vi "test-cubic-spline-04A.vi"() -> (3 "Test Passed":bool)   [LabVIEW 2019]
uses:
  <vilib>/Rock Robotics/WPI/ThirdParty/JAS_Junk/TrajLib/POSEwCURVATURE.ctl
  <vilib>/Rock Robotics/WPI/ThirdParty/JAS_Junk/TrajLib/POSE2D.ctl
  <vilib>/Rock Robotics/WPI/ThirdParty/JAS_Junk/TrajLib/TRANSLATION2D.ctl
  <vilib>/Rock Robotics/WPI/ThirdParty/JAS_Junk/TrajLib/ROTATION2D.ctl
  <vilib>/Rock Robotics/WPI/ThirdParty/JAS_Junk/TrajLib/Rotation_CreateAngle.vi
  <vilib>/Rock Robotics/WPI/ThirdParty/JAS_Junk/TrajLib/Translation_Create.vi
  <vilib>/Rock Robotics/WPI/ThirdParty/JAS_Junk/TrajLib/Util_CalcDist.vi
  <vilib>/Rock Robotics/WPI/ThirdParty/JAS_Junk/TrajLib/Trajectory_Library.lvlib
panel:
  out "XY Graph":cluster{dbl[], dbl[]}(graph)
  out "All Interior \nwayPoints\nFound (True)":bool
  out "end rot = 0":dbl
  out "end y = 0":dbl
  out "end x = 0":dbl
  out "start rot = 0":dbl
  out "start y = 0":dbl
  out "start x = 0":dbl
  out "max dtheta < 0.0872":dbl
  out "max dy < 0.00127":dbl
  out "max dx  < 0.127":dbl
  out "Overall Error":errorcluster
  out "Elements":i32
  out "Create Spline Error":errorcluster
  out "SplinePoses\nWCurve":T1[](array[typedef]) {"POSE"."ROTATION"."SIN" format="%13.4f"; "POSE"."ROTATION"."COS" format="%13.4f"; "POSE"."ROTATION"."VALUE" format="%13.4f"; "POSE"."TRANSLATION"."Y" format="%14.3f"; "POSE"."TRANSLATION"."X" format="%14.3f"}
  out "Elapsed Time":dbl
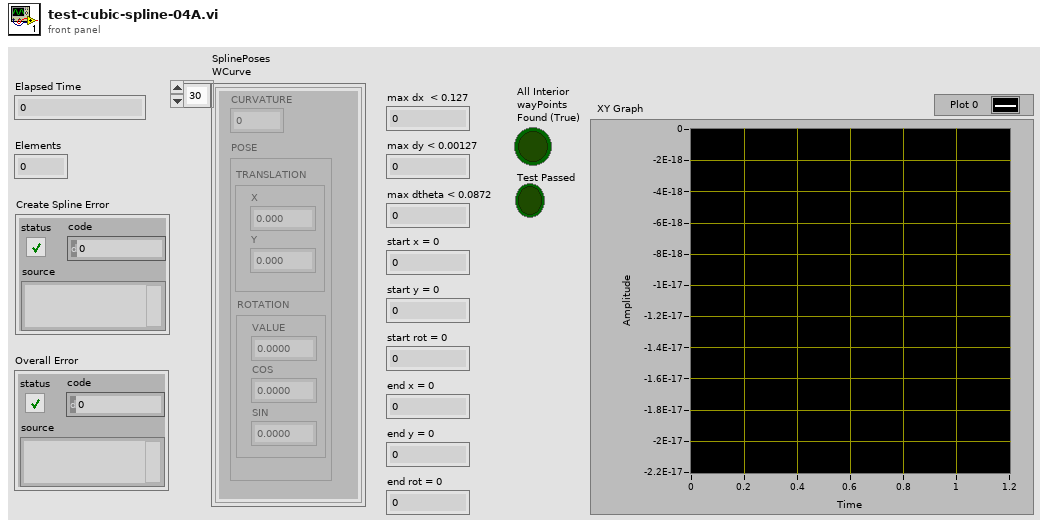
[diagram p1: front panel]
types:
  T1 = typedef "Trajectory_Library.lvlib/POSEwCURVATURE.ctl" = cluster{"CURVATURE":dbl, "POSE":T2}
  T2 = typedef "Trajectory_Library.lvlib/POSE2D.ctl" = cluster{"TRANSLATION":T3, "ROTATION":T4}
  T3 = typedef "Trajectory_Library.lvlib/TRANSLATION2D.ctl" = cluster{"X":dbl, "Y":dbl}
  T4 = typedef "Trajectory_Library.lvlib/ROTATION2D.ctl" = cluster{"VALUE":dbl, "COS":dbl, "SIN":dbl}
  T5 = typedef "Trajectory_Library.lvlib/SPLINE_CTRL_VECTOR.ctl" = cluster{"Xs":dbl[], "Ys":dbl[]}
  T6 = typedef "Trajectory_Library.lvlib/SPLINE.ctl" = cluster{"Degree":i32, "Coefficients":T7}
  T7 = typedef "NI_Matrix.lvlib/RealMatrix.ctl" = dbl[][]
  T8 = typedef "Trajectory_Library.lvlib/TWIST2D.ctl" = cluster{"dX":dbl, "dY":dbl, "dTHETA":dbl}
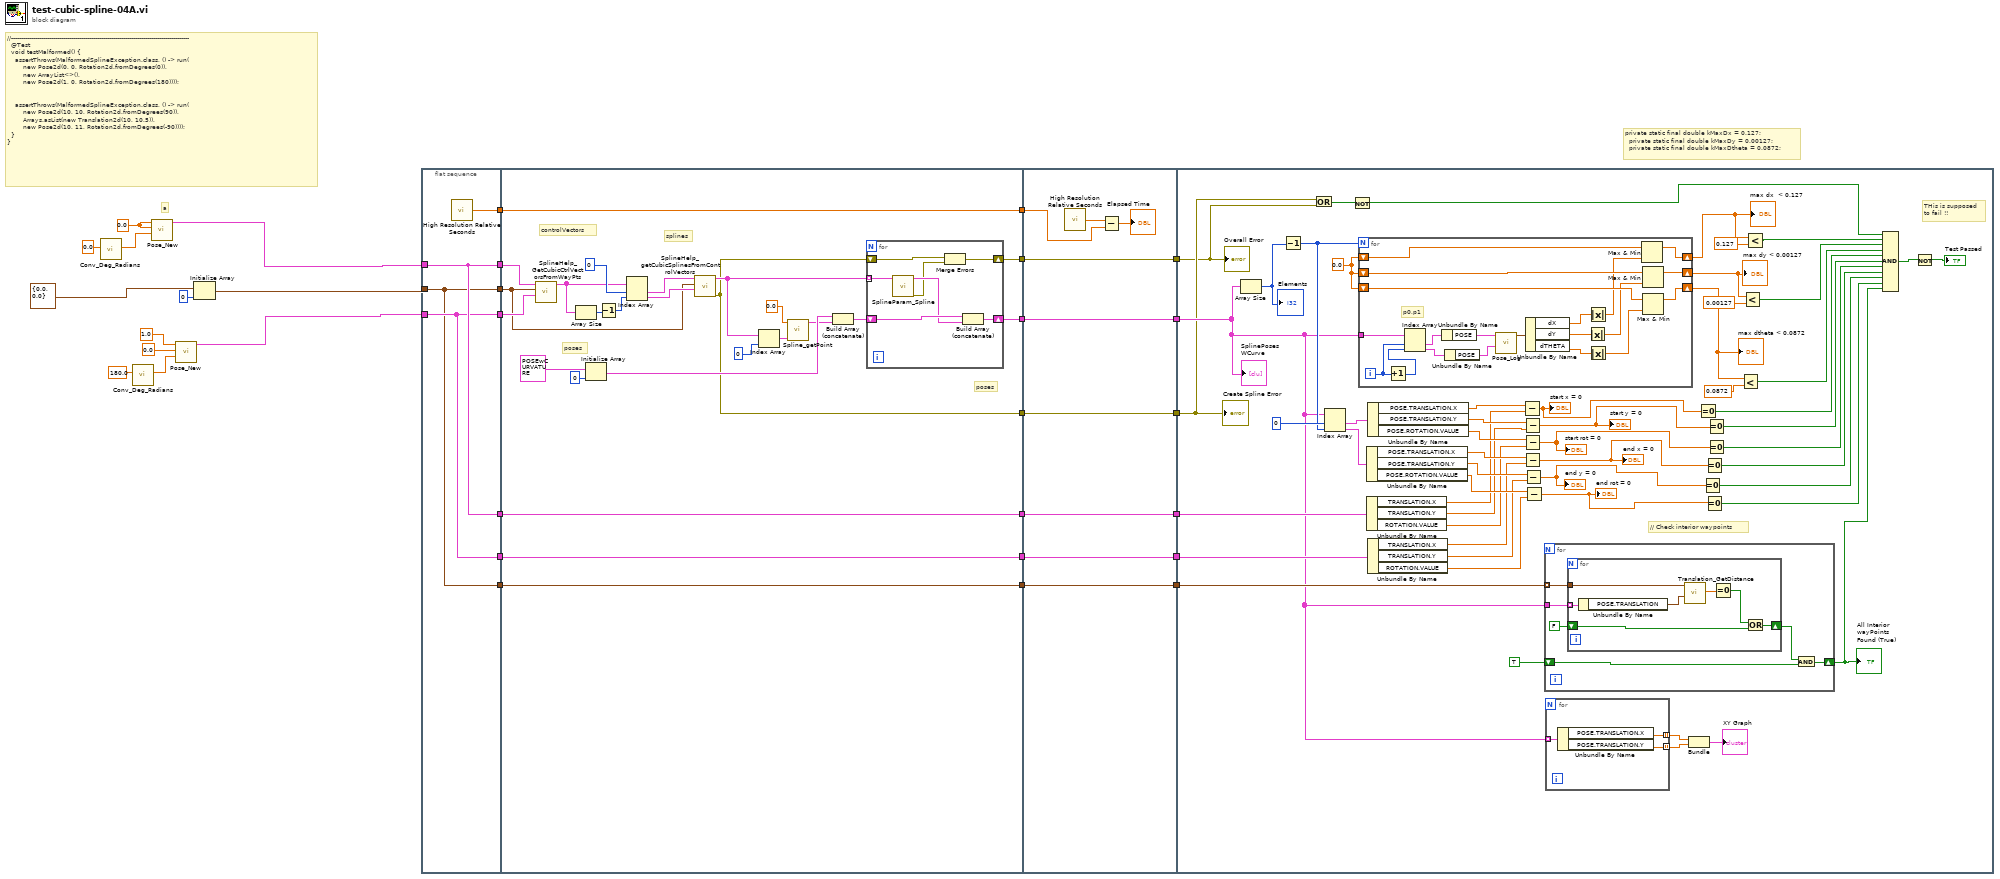
[diagram p0: block diagram]
diagram:
  w10 = 0.0 ("X")
  # "a"
  # "//-----------------------------------------------------------------------------------------\n  @Test\n  void testMalformed() {\n    assertThrows(MalformedSplineException.class, () -> run(\n        new Pose2d(0, 0, Rotation2d.fromDegrees(0)),\n        new ArrayList<>(), \n        new Pose2d(1, 0, Rotation2d.fromDegrees(180))));\n\n\n    assertThrows(MalformedSplineException.class, () -> run(\n        new Pose2d(10, 10, Rotation2d.fromDegrees(90)),\n        Arrays.asList(new Translation2d(10, 10.5)),\n        new Pose2d(10, 11, Rotation2d.fromDegrees(-90))));\n  }\n}"
  # "private static final double kMaxDx = 0.127;\n  private static final double kMaxDy = 0.00127;\n  private static final double kMaxDtheta = 0.0872;"
  n1 = call <vilib>:"Conv_Deg_Radians.vi"("Degress"=0.0) -> ("Radians"=w9:dbl)  [unwired: 10 in]
  n2 = call <vilib>:"Conv_Deg_Radians.vi"("Degress"=180.0) -> ("Radians"=w6:dbl)  [unwired: 10 in]
  n3 = call <vilib>:"Pose_New.vi"("Heading"=w9, "Y"=w10, "X"=w10) -> ("out POSe"=w3:T2)  [unwired: 8 in]
  n4 = call <vilib>:"Pose_New.vi"("Heading"=w6, "Y"=0.0, "X"=1.0) -> ("out POSe"=w1:T2)  [unwired: 8 in]
  n5 = Initialize Array(T3 {"X"=0.0, "Y"=0.0} ("TRANSLATION"), 0 ("dimension size")) -> (w2:T3[])
  n6 = flat-sequence {
    tunnel: w3 -> [w35]
    tunnel: [w35] -> w32
    tunnel: w2 -> [w33]
    tunnel: [w33] -> w31
    tunnel: w1 -> [w34]
    tunnel: [w34] -> w30
    tunnel: [w36] -> w29
    tunnel: [w35] -> w21
    tunnel: [w34] -> w18
    tunnel: [w33] -> w13
    tunnel: w32 -> [w61]
    tunnel: w31 -> [w53]
    tunnel: w30 -> [w60]
    tunnel: [w52] -> w28
    tunnel: w29 -> [w52]
    tunnel: [w42] -> w27
    tunnel: [w41] -> w25
    tunnel: [w40] -> w23
    tunnel: w21 -> [w39]
    tunnel: [w39] -> w20
    tunnel: w18 -> [w38]
    tunnel: [w38] -> w17
    tunnel: [w37] -> w14
    tunnel: w13 -> [w37]
    tunnel: w28 -> [w77]
    tunnel: w27 -> [w76]
    tunnel: [w76] -> w26
    tunnel: w25 -> [w75]
    tunnel: [w75] -> w24
    tunnel: w23 -> [w74]
    tunnel: [w74] -> w22
    tunnel: w20 -> [w71]
    tunnel: [w71] -> w19
    tunnel: w17 -> [w70]
    tunnel: [w70] -> w16
    tunnel: [w69] -> w15
    tunnel: w14 -> [w69]
    tunnel: w26 -> [w106]
    tunnel: w24 -> [w82]
    tunnel: w22 -> [w81]
    tunnel: w19 -> [w129]
    tunnel: w16 -> [w128]
    tunnel: w15 -> [w111]
    frame #0 {
      n7 = call <vilib>:"High Resolution Relative Seconds.vi"() -> ("relative seconds"=w36:dbl)
    }
    frame #1 {
      # "poses"
      # "poses"
      # "splines"
      # "controlVectors"
      n8 = call <vilib>:"SplineHelp_GetCubicCtrlVectorsFromWayPts.vi"("Enging POSE"=w60, "Interior WAYPOINTS"=w53, "Starting POSE"=w61) -> ("SplineControlVectors"=w57:T5[])  [unwired: 8 in]
      n9 = Array Size(array=w57) -> (size(s)=w58:i32)
      n10 = Initialize Array(T1 {"CURVATURE"=0.0, "POSE"={"TRANSLATION"={"X"=0.0, "Y"=0.0}, "ROTATION"={"VALUE"=0.0, "COS"=1.0, "SIN"=0.0}}} ("POSEwCURVATURE"), 0 ("dimension size")) -> (w46:T1[])
      n11 = Decrement(x=w58) -> (x-1=w56:i32)
      n12 = Index Array(array=w57, index #1=0 ("index"), index #2=w56) -> (element #1=w55:T5, element #2=w54:T5)
      n13 = call <vilib>:"SplineHelp_getCubicSplinesFromControlVectors.vi"("endCtrlVector"=w54, "InternalWaypoints"=w53, "startCtrlVector"=w55) -> ("error out"=w41:errorcluster, "splines"=w43:T6[])  [unwired: 3 in, 4 out]
      n14 = Index Array(array=w43, index=0) -> (element=w48:T6)
      n15 = call <vilib>:"Spline_getPoint.vi"("inputSPLINE"=w48, "Time"=0.0) -> ("POSEwCURVATURE"=w45:T1)  [unwired: 9 in]
      n16 = Build Array (concatenate)(w46, w45) -> (w44:T1[])
      n17 = for {
        shift-right: [w65] -> w42
        shift-left: w44 -> [w67]
        tunnel: w43 -> [w68] mode=indexing
        shift-right: [w63] -> w40
        shift-left: w41 -> [w64]
        n18 = call <vilib>:"SplineParam_Spline.vi"("inputSPLINE"=w68) -> ("error out"=w62:errorcluster, "outputPOSEwCURVATURE"=w66:T1[])  [unwired: 9 in]
        n19 = Merge Errors(w64, w62) -> (w63:errorcluster)
        n20 = Build Array (concatenate)(w67, w66) -> (w65:T1[])
      }
    }
    frame #2 {
      n21 = call <vilib>:"High Resolution Relative Seconds.vi"() -> ("relative seconds"=w72:dbl)
      n22 = Subtract(x=w72, y=w77) -> (x-y=→"Elapsed Time":dbl)
    }
    frame #3 {
      w130 = 0.0
      # "THis is supposed\nto fail !!"
      # "// Check interior waypoints"
      n23 = Array Size(array=w106) -> (size(s)=w131:i32)
      "Elements" <- w131
      n24 = Decrement(x=w131) -> (x-1=w126:i32)
      n25 = Or(x=w82, y=w81) -> (x .or. y?=w83:bool)
      n26 = Index Array(array=w106, index #1=0 ("index"), index #2=w126) -> (element #1=w125:T1, element #2=w124:T1)
      n27 = Not(x=w83) -> (.not. x?=w80:bool)
      n28 = for {
        N: w126 -> [_]
        tunnel: w106 -> [w165]
        shift-right: [w156] -> w103
        shift-left: w130 -> [w153]
        shift-right: [w154] -> w105
        shift-left: w130 -> [w151]
        shift-right: [w155] -> w104
        shift-left: w130 -> [w152]
        i -> [w167]
        # "p0,p1"
        n29 = Increment(x=w167) -> (x+1=w166:i32)
        n30 = Index Array(array=w165, index #1=w167, index #2=w166) -> (element #1=w164:T1, element #2=w163:T1)
        n31 = Unbundle By Name(w164) -> ("POSE"=w162:T2)
        n32 = Unbundle By Name(w163) -> ("POSE"=w161:T2)
        n33 = call <vilib>:"Pose_Log.vi"("end POSE"=w161, "in POSE"=w162) -> ("out TWIST"=w160:T8)  [unwired: 9 in]
        n34 = Unbundle By Name(w160) -> ("dX"=w157:dbl, "dY"=w158:dbl, "dTHETA"=w159:dbl)
        n35 = Absolute Value(x=w158) -> (abs(x)=w149:dbl)
        n36 = Absolute Value(x=w157) -> (abs(x)=w150:dbl)
        n37 = Absolute Value(x=w159) -> (abs(x)=w148:dbl)
        n38 = Max & Min(x=w153, y=w150) -> (max(x,y)=w156:dbl)  [unwired: 1 out]
        n39 = Max & Min(x=w152, y=w149) -> (max(x,y)=w155:dbl)  [unwired: 1 out]
        n40 = Max & Min(x=w151, y=w148) -> (max(x,y)=w154:dbl)  [unwired: 1 out]
      }
      "max dx  < 0.127" <- w103
      "max dy < 0.00127" <- w104
      "max dtheta < 0.0872" <- w105
      n41 = Unbundle By Name(w124) -> ("POSE.TRANSLATION.X"=w120:dbl, "POSE.TRANSLATION.Y"=w119:dbl, "POSE.ROTATION.VALUE"=w118:dbl)
      n42 = Unbundle By Name(w129) -> ("TRANSLATION.X"=w117:dbl, "TRANSLATION.Y"=w116:dbl, "ROTATION.VALUE"=w115:dbl)
      n43 = Unbundle By Name(w125) -> ("POSE.TRANSLATION.X"=w123:dbl, "POSE.TRANSLATION.Y"=w122:dbl, "POSE.ROTATION.VALUE"=w121:dbl)
      n44 = Unbundle By Name(w128) -> ("TRANSLATION.X"=w114:dbl, "TRANSLATION.Y"=w113:dbl, "ROTATION.VALUE"=w112:dbl)
      n45 = Subtract(x=w123, y=w117) -> (x-y=w96:dbl)
      "start x = 0" <- w96
      n46 = Subtract(x=w122, y=w116) -> (x-y=w95:dbl)
      "start y = 0" <- w95
      n47 = Subtract(x=w121, y=w115) -> (x-y=w94:dbl)
      "start rot = 0" <- w94
      n48 = Subtract(x=w120, y=w114) -> (x-y=w93:dbl)
      "end x = 0" <- w93
      n49 = Subtract(x=w119, y=w113) -> (x-y=w92:dbl)
      "end y = 0" <- w92
      n50 = Subtract(x=w118, y=w112) -> (x-y=w91:dbl)
      "end rot = 0" <- w91
      n51 = for {
        tunnel: w111 -> [w135] mode=indexing
        tunnel: w106 -> [w140]
        shift-right: [w139] -> w84
        shift-left: TRUE -> [w138]
        n52 = for {
          tunnel: w140 -> [w144] mode=indexing
          shift-right: [w147] -> w136
          shift-left: FALSE -> [w146]
          tunnel: w135 -> [w145]
          n53 = Unbundle By Name(w144) -> ("POSE.TRANSLATION"=w143:T3)
          n54 = call <vilib>:"Translation_GetDistance.vi"("other Translation"=w143, "In Translation"=w145) -> ("Distance"=w142:dbl)  [unwired: 9 in]
          n55 = Equal To 0?(x=w142) -> (x = 0?=w141:bool)
          n56 = Or(x=w141, y=w146) -> (x .or. y?=w147:bool)
        }
        n57 = And(x=w136, y=w138) -> (x .and. y?=w139:bool)
      }
      "All Interior \nwayPoints\nFound (True)" <- w84
      n58 = for {
        tunnel: [w134] -> w109 mode=indexing
        tunnel: [w133] -> w108 mode=indexing
        tunnel: w106 -> [w132] mode=indexing
        n59 = Unbundle By Name(w132) -> ("POSE.TRANSLATION.X"=w134:dbl, "POSE.TRANSLATION.Y"=w133:dbl)
      }
      n60 = Bundle(w109, w108) -> (→"XY Graph":cluster{dbl[], dbl[]})  [unwired: 1 in]
      n61 = Equal To 0?(x=w96) -> (x = 0?=w90:bool)
      n62 = Equal To 0?(x=w92) -> (x = 0?=w86:bool)
      n63 = Equal To 0?(x=w93) -> (x = 0?=w87:bool)
      n64 = Equal To 0?(x=w91) -> (x = 0?=w85:bool)
      n65 = Equal To 0?(x=w95) -> (x = 0?=w89:bool)
      n66 = Equal To 0?(x=w94) -> (x = 0?=w88:bool)
      n67 = Less?(x=w105, y=0.0872) -> (x < y?=w97:bool)
      n68 = Less?(x=w104, y=0.00127) -> (x < y?=w98:bool)
      n69 = Less?(x=w103, y=0.127) -> (x < y?=w99:bool)
      n70 = Compound Arithmetic op=AND(w80, w99, w98, w97, w90, w89, w88, w87, w86, w85, w84) -> (w78:bool)
      n71 = Not(x=w78) -> (.not. x?=→"Test Passed":bool)
      "SplinePoses\nWCurve" <- w106
      "Create Spline Error" <- w82
      "Overall Error" <- w81
    }
  }
